vi "Serial Loopback Test.vi"() -> ()   [LabVIEW 2025]
doc: "This example shows how to do basic serial loopback test. It is a convenient way to test if a serial port is working.\n\nThis example works with the Onboard RS-232 port on the roboRIO, or with the MXP UART port on the roboRIO.\n\nNote: before using this example with RS-232 you must turn off Console Out on the roboRIO. This can be done in the roboRIO Imaging Tool.\n\nTo use this example:\n1. Choose the Serial Port: either MXP TTL or Onboard RS-232\n2. Connect loopback wiring: RX to TX for MXP TTL, or RXD to TXD for Onboard RS-232\n3. Run the example, type into the 'Text to Write' control, and press the Write button\n4. Your text should appear in the 'Loopback Read' indicator"
uses:
  <vilib>/Rock Robotics/WPI/SerialPort/WPI_SerialPort.ctl
panel:
  out "Loopback Read":string
  in  "Serial Port":T1=enum."MXP TTL"
  in  "write":bool
  in  "stop":bool
  out "Bytes Written":u32
  in  "Text to Write":string="Testing FRC serial write message. Can you read it?"
  in  "Flow Control":u16(ring) items=["None", "XON/XOFF", "RTS/CTS", "XON/XOFF & RTS/CTS", "DTR/DSR", "XON/XOFF & DTR/DSR"]
  in  "Stop Bits":u16(ring)=10 items=["1.0"=10, "1.5"=15, "2.0"=20]
  in  "Parity":u16(ring) items=["None", "Odd", "Even", "Mark", "Space"]
  in  "Data Bits":u16=8
  in  "Baud Rate":u32=115200
  # "Set these inputs before running."
  # "Controls and Output"
  # "Connect loopback wiring according to the Serial Port control value."
  # "RS-232\nconnect RXD to TXD\n\nUART\nconnect MXP RX to MXP TX\n(MXP pin 10 to pin 14)"
  # "Note: before using this example with RS-232 you must turn off Console Out on the roboRIO.  This can be done in the roboRIO Imaging Tool"
  # "This shows wiring for serial communication loop back testing."
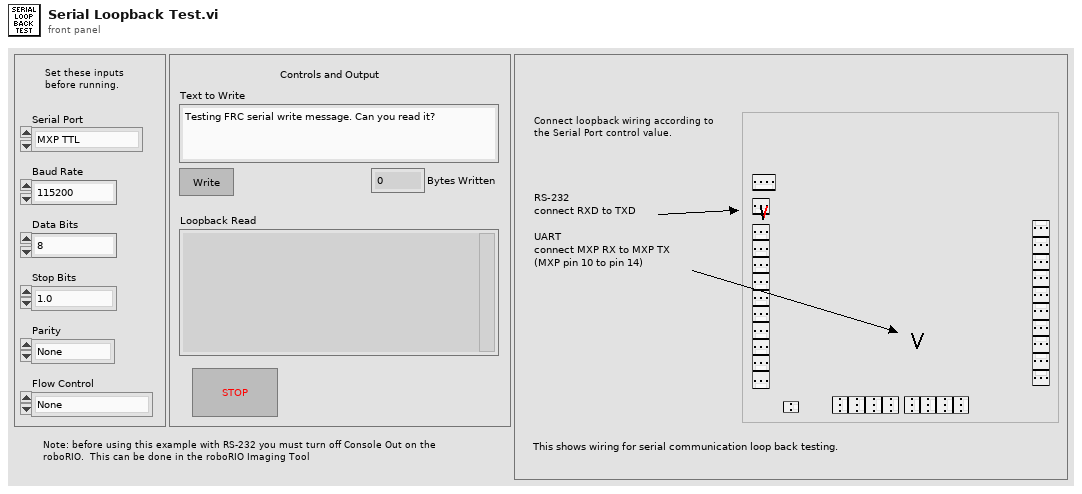
[diagram p1: front panel]
types:
  T1 = typedef "WPI_SerialPort.ctl" = enum16{"Onboard RS-232", "MXP TTL", "USB 1", "USB 2"}
  T2 = typedef "WPI_SerialPortRef.ctl" = cluster{"DevStatus":errorcluster, "Serial Port Name":refnum<visa-resource-name>}
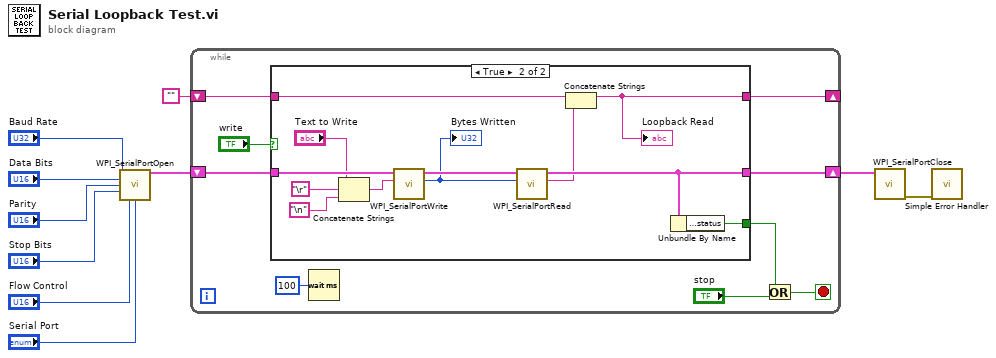
[diagram p0: block diagram]
diagram:
  n1 = call <vilib>:"WPI_SerialPortOpen.vi"("Baud Rate"="Baud Rate", "Data Bits"="Data Bits", "Parity"="Parity", "Stop Bits"="Stop Bits", "Flow Control"="Flow Control", "Serial Port"="Serial Port") -> ("SerialPortRef"=w6:T2)  [unwired: 8 in, 1 out]
  n2 = while {
    shift-right: [w17] -> w5
    shift-left: w6 -> [w19]
    shift-right: [w11] -> _
    shift-left: "" -> [w12]
    stop <- w16 stop-if-true
    n3 = case shown="True" "write" {
      tunnel: w19 -> [w21 w33]
      tunnel: [w21 w26] -> w17
      tunnel: [_ w29] -> w13
      tunnel: w12 -> [w20 w24]
      tunnel: [w20 w22] -> w11
      frame False {
      }
      frame True {
        n4 = Concatenate Strings("Text to Write", "\r", "\n") -> (w30:string)
        n5 = call <vilib>:"WPI_SerialPortWrite.vi"("Buffer"=w30, "SerialPortRef"=w33) -> ("Num Bytes Written"=w25:u32, "SerialPortRef"=w27:T2)  [unwired: 7 in, 1 out]
        "Bytes Written" <- w25
        n6 = call <vilib>:"WPI_SerialPortRead.vi"("Num Bytes to Read"=w25, "SerialPortRef"=w27) -> ("Buffer"=w23:string, "SerialPortRef"=w26:T2)  [unwired: 7 in, 1 out]
        n7 = Concatenate Strings(w24, w23) -> (w22:string)
        "Loopback Read" <- w22
        n8 = Unbundle By Name(w26) -> ("DevStatus.status"=w29:bool)
      }
    }
    n9 = Wait (ms)(milliseconds to wait=u32 100) -> ()  [unwired: 1 out]
    n10 = Or(x=w13, y="stop") -> (x .or. y?=w16:bool)
  }
  n11 = call <vilib>:"WPI_SerialPortClose.vi"("SerialPortRef"=w5) -> ("error out"=w3:errorcluster)  [unwired: 10 in]
  n12 = call <vilib>:"Simple Error Handler.vi"("error in (no error)"=w3) -> ()  [unwired: 4 in, 5 out]
